vi "Read Library Name.vi"(8 "error in (no error)":errorcluster, 11 "Library in":refnum<class "Library.lvclass">) -> (0 "error out":errorcluster, 2 "Library Name":string, 3 "Library out":refnum<class "Library.lvclass">)   [LabVIEW 2019, in "Panther Dashboard.lvlib" / "Library.lvclass"]
uses:
  Library.lvclass
  Library.lvclass/Library.ctl
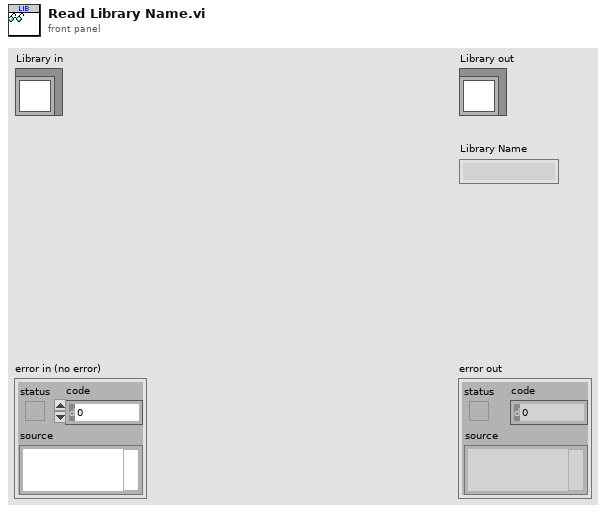
[diagram p1: front panel]
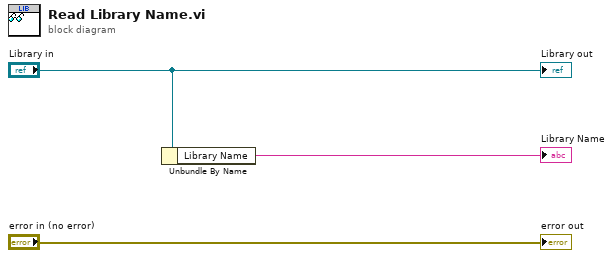
[diagram p0: block diagram]
diagram:
  n1 = Unbundle By Name("Library in") -> ("Library Name"=→"Library Name":string)
  "error out" <- "error in (no error)"
  "Library out" <- "Library in"
